vi "Gen_3D_pattern.vi"(0 "X: fast axis":T3, 1 "asymmetry":dbl=0.9, 3 "Home the stage after scan?":bool, 5 "Y: points":T2, 9 "Z: points":T2, 10 "Soften":bool, 11 "error in (no error)":errorcluster, 12 "Scan mode":T1(ring)=enum."Single Direction (Uniform)", 13 "Soften points":i32=3, 14 "Lissajous Cluster":cluster{"a":dbl, "b":dbl, "delta":dbl}={"a"=1.0, "b"=2.0, "delta"=0.0} {"delta" format="%_3g"; "b" format="%0.2p"; "a" format="%_3g"}) -> (4 "Samples per channel":i32, 6 "Scan pattern":dbl[][](graph), 15 "error out":errorcluster)   [LabVIEW 2014]
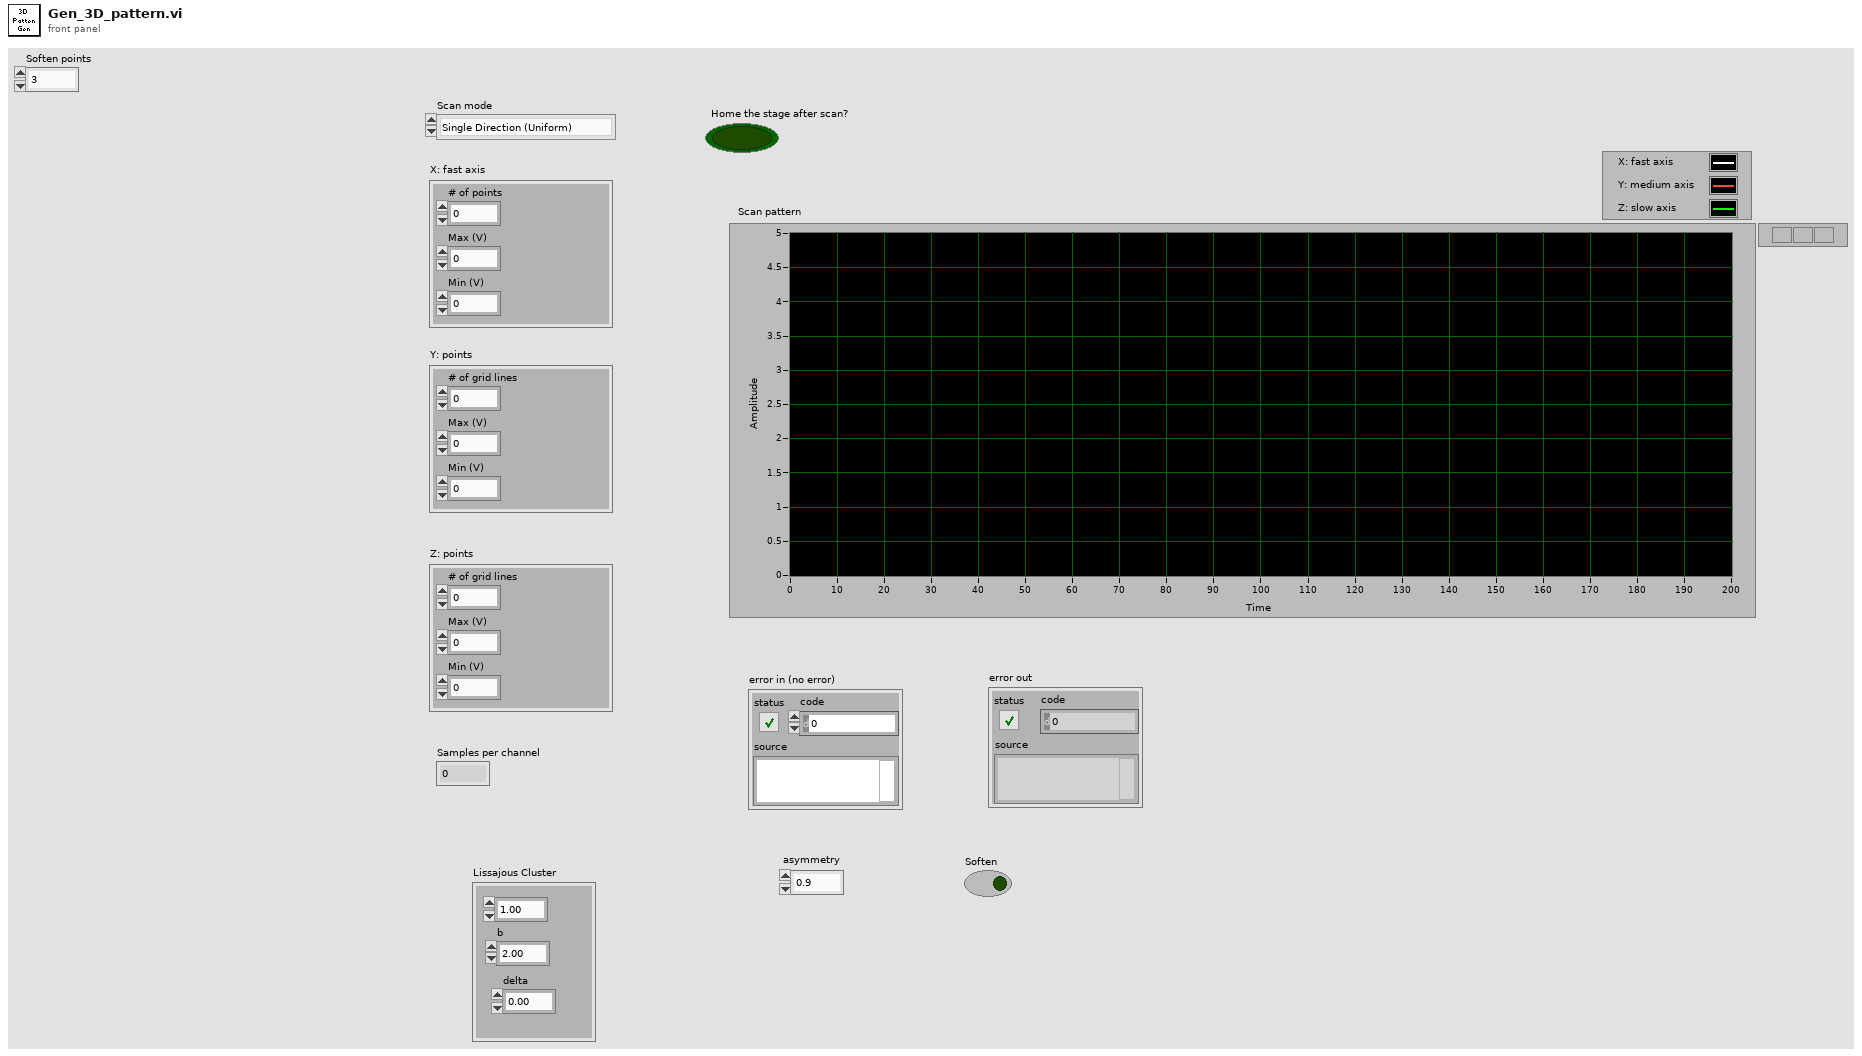
[diagram p1: front panel]
types:
  T1 = enum16{"Lissajous", "Adjustable sawtooth", "Single Direction (Uniform)", "Single Direction (Fast Reset)", "Bi-Directional"}
  T2 = cluster{"# of grid lines":u16, "Max (V)":dbl, "Min (V)":dbl}
  T3 = cluster{"# of points":u16, "Max (V)":dbl, "Min (V)":dbl}
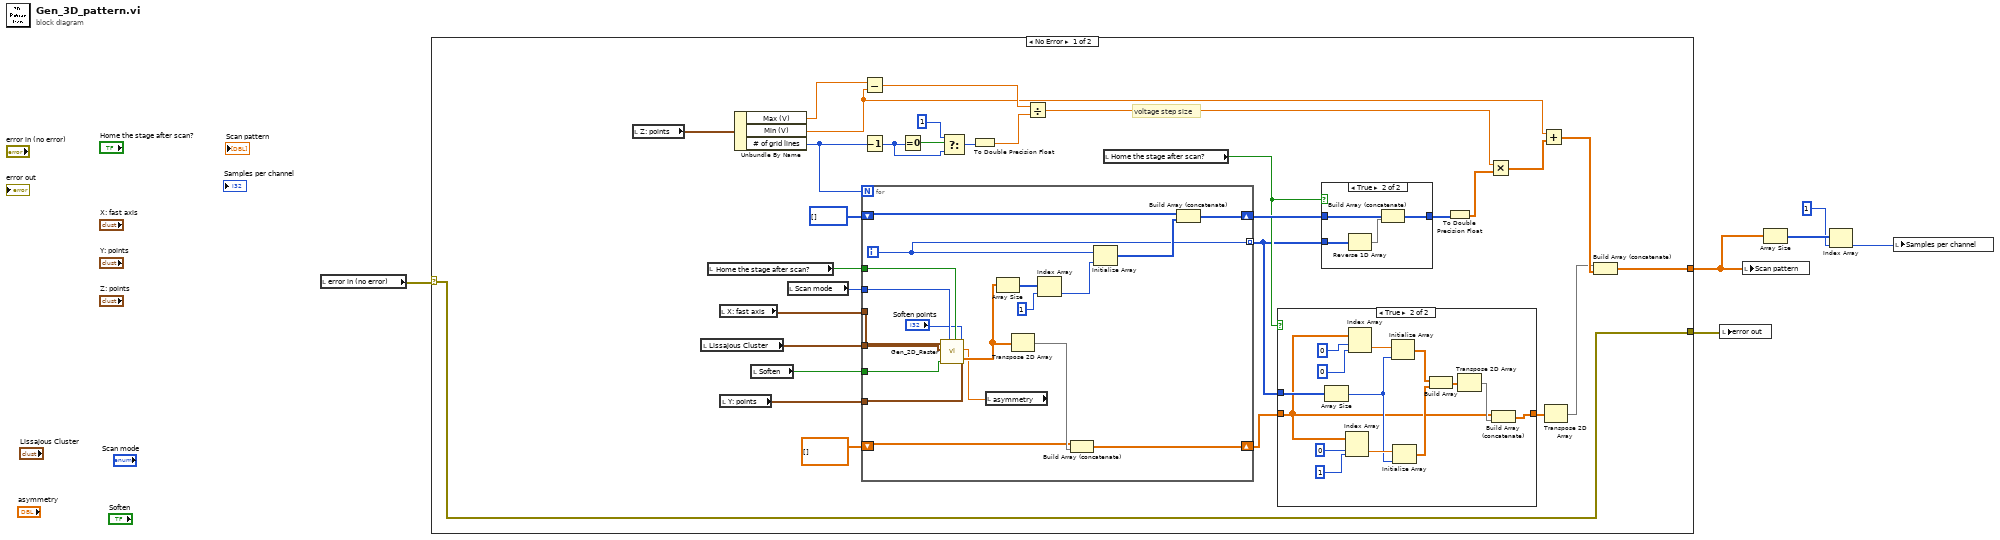
[diagram p0: block diagram]
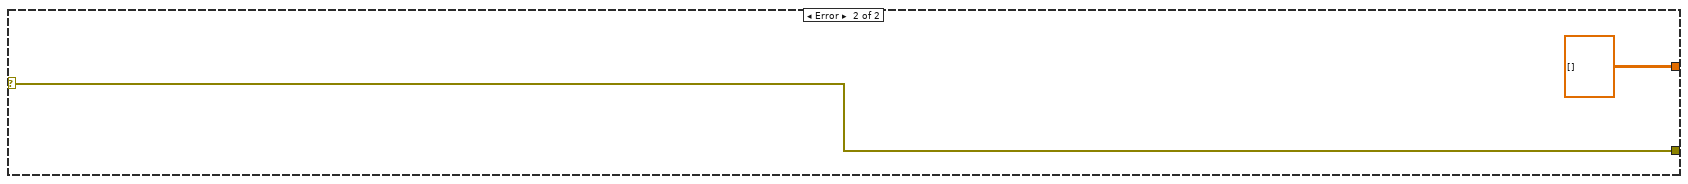
[diagram p4: hidden frame]
diagram:
  n1 = local read "error in (no error)"() -> (w6:errorcluster)
  n2 = case shown="No Error" w6 {
    selector: w6 -> [w20 w78]
    tunnel: [w20 w78] -> w5
    tunnel: [w18 dbl[][] []] -> w4
    frame No Error {
      # "voltage step size"
      n3 = local read "Z: points"() -> (w37:T2)
      n4 = local read "Lissajous Cluster"() -> (w8:cluster{"a":dbl, "b":dbl, "delta":dbl})
      n5 = local read "Home the stage after scan?"() -> (w15:bool)
      n6 = local read "X: fast axis"() -> (w10:T3)
      n7 = local read "Y: points"() -> (w9:T2)
      n8 = Unbundle By Name(w37) -> ("Max (V)"=w35:dbl, "Min (V)"=w28:dbl, "# of grid lines"=w36:u16)
      n9 = local read "Soften"() -> (w7:bool)
      n10 = local read "Scan mode"() -> (w21:T1)
      n11 = for {
        N: w36 -> [_]
        tunnel: w10 -> [w63]
        tunnel: w9 -> [w62]
        shift-right: [w74] -> w11
        shift-left: dbl[][] [] -> [w75]
        shift-right: [w73] -> w17
        shift-left: i8[] [] -> [w72]
        tunnel: w21 -> [w66]
        tunnel: w15 -> [w65]
        tunnel: [w64] -> w12 mode=indexing
        tunnel: w8 -> [w61]
        tunnel: w7 -> [w60]
        i -> [w64]
        n12 = local read "asymmetry"() -> (w59:dbl)
        n13 = call "Gen_2D_Raster.vi"("Fast-axis Para"=w63, "Lissajous Cluster"=w61, "Soften"=w60, "Pattern"=w66, "Reset slow axis at End of Scan?"=w65, "asymmetry"=w59, "Soften points"="Soften points", "Slow-axis Para"=w62) -> ("2D Raster Pattern"=w67:dbl[][])  [unwired: 1 in, 1 out]
        n14 = Array Size(array=w67) -> (size(s)=w69:i32[])
        n15 = Transpose 2D Array(2D array=w67) -> (transposed array=w76:dbl[][])
        n16 = Index Array(array=w69, index=1) -> (element=w68:i32)
        n17 = Build Array (concatenate)(w75, w76) -> (w74:dbl[][])
        n18 = Initialize Array(w64, w68) -> (w71:i32[])
        n19 = Build Array (concatenate)(w72, w71) -> (w73:i32[])
      }
      n20 = Decrement(x=w36) -> (x-1=w24:u16)
      n21 = Subtract(x=w35, y=w28) -> (x-y=w34:dbl)
      n22 = Equal To 0?(x=w24) -> (x = 0?=w26:bool)
      n23 = Select(t=1, s=w26, f=w24) -> (s? t:f=w23:i32)
      n24 = To Double Precision Float(number=w23) -> (double precision float=w22:dbl)
      n25 = Divide(x=w34, y=w22) -> (x/y=w30:dbl)
      n26 = local read "Home the stage after scan?"() -> (w14:bool)
      n27 = case shown="True" w14 {
        tunnel: w11 -> [w38 w39]
        tunnel: [w38 w41] -> w13
        tunnel: w12 -> [_ w47]
        frame False {
        }
        frame True {
          n28 = Array Size(array=w47) -> (size(s)=w45:i32)
          n29 = Index Array(array=w39, index (row)=0, index (col)=1) -> (element=w46:dbl)
          n30 = Index Array(array=w39, index (row)=0, index (col)=0) -> (element=w48:dbl)
          n31 = Initialize Array(w48, w45) -> (w44:dbl[])
          n32 = Initialize Array(w46, w45) -> (w43:dbl[])
          n33 = Build Array(w44, w43) -> (w42:dbl[][])
          n34 = Transpose 2D Array(2D array=w42) -> (transposed array=w40:dbl[][])
          n35 = Build Array (concatenate)(w39, w40) -> (w41:dbl[][])
        }
      }
      n36 = case shown="True" w14 {
        tunnel: w17 -> [w53 w56]
        tunnel: [w53 w54] -> w16
        tunnel: w12 -> [_ w57]
        frame False {
        }
        frame True {
          n37 = Reverse 1D Array(array=w57) -> (reversed array=w55:i32[])
          n38 = Build Array (concatenate)(w56, w55) -> (w54:i32[])
        }
      }
      n39 = To Double Precision Float(number=w16) -> (double precision float=w31:dbl[])
      n40 = Multiply(x=w30, y=w31) -> (x*y=w29:dbl[])
      n41 = Add(x=w28, y=w29) -> (x+y=w27:dbl[])
      n42 = Transpose 2D Array(2D array=w13) -> (transposed array=w19:dbl[][])
      n43 = Build Array (concatenate)(w19, w27) -> (w18:dbl[][])
    }
    frame Error {
    }
  }
  n44 = local write "error out"(w5) -> ()
  n45 = local write "Scan pattern"(w4) -> ()
  n46 = Array Size(array=w4) -> (size(s)=w3:i32[])
  n47 = Index Array(array=w3, index=u8 1) -> (element=w1:i32)
  n48 = local write "Samples per channel"(w1) -> ()
